vi "_Release CSMQ.vi"(8 "Error in":errorcluster caption="Error in (no error)", 11 "CSMQ":T1) -> (0 "Error out":errorcluster)   [LabVIEW 2014, in "Communicable State Machine.lvlib"]
uses:
  Communicable State Machine.lvlib
  _CSMQ.ctl
  Typedef/_Cross JKISM State Data.ctl
  Typedef/_CSM_MSG_TYPE.ctl
  Typedef/_Cross JKISM State Response.ctl
  Typedef/_CSM_MODE.ctl
  Typedef/_CSM Status Change Event Data.ctl
  _CSMQFGVOPER.ctl
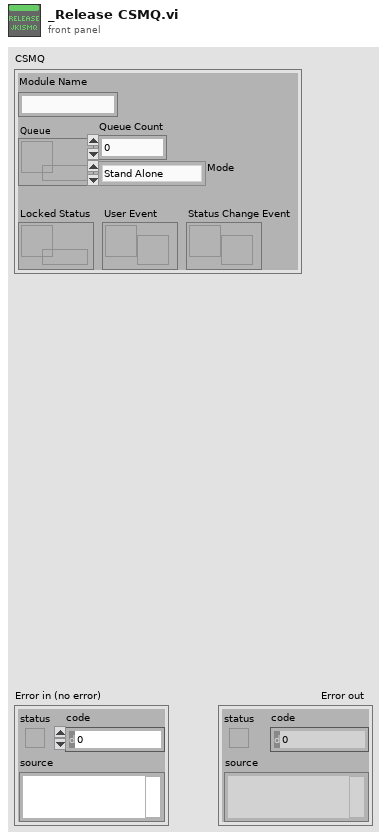
[diagram p1: front panel]
types:
  T1 = typedef "Communicable State Machine.lvlib/_CSMQ.ctl" = cluster{"Module Name":string, "Queue":refnum<queue>, "Locked Status":refnum<data-value>, "Mode":T2, "User Event":refnum<user-event>, "Queue Count":i32, "Status Change Event":refnum<user-event>}
  T2 = typedef "Communicable State Machine.lvlib/_CSM_MODE.ctl" = enum16{"Stand Alone", "JKISM", "Action Worker"}
  T3 = typedef "Communicable State Machine.lvlib/_CSMQFGVOPER.ctl" = enum16{"Get By Name", "List", "Check If Name Exists", "Release", "Module Status", "Create Status Event Handler", "Destroy Status Event Handler"}
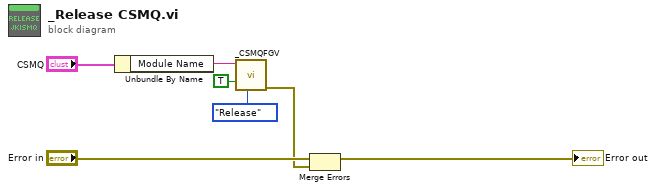
[diagram p0: block diagram]
diagram:
  n1 = Unbundle By Name("CSMQ") -> ("Module Name"=w5:string)
  n2 = call "_CSMQFGV.vi"("Operation"=_CSMQFGVOPER."Release", "create if not found? (T)"=TRUE, "Name(\"\" to use uuid) in"=w5) -> ("Error out"=w2:errorcluster)  [unwired: 5 in, 3 out]
  n3 = Merge Errors("Error in", w2) -> (→"Error out":errorcluster)
